vi "Wilcoxon Signed Rank Test.vi"   [LabVIEW 2012, in "NI_Gmath.lvlib"]
doc: "Tests hypotheses about the <B>mean</B> of populations whose distributions are continuous and symmetric but not necessarily normal. You must manually select the polymorphic instance to use."
uses:
  NI_Gmath.lvlib
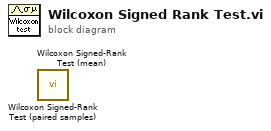
[diagram p0: block diagram]
diagram:
  n1 = call "Wilcoxon Signed-Rank Test (paired samples).vi"() -> ()  [unwired: 9 in, 3 out]
  n2 = call "Wilcoxon Signed-Rank Test (mean).vi"() -> ()  [unwired: 9 in, 3 out]
